vi "rs3 Advanced get color correction3.vi"(8 "error in (no error)":errorcluster, 10 "mode":i32, 11 "device in":u64) -> (0 "error out 2":errorcluster, 1 "error":u64, 2 "STColorCorrection output":T1, 3 "Dev out":u64)   [LabVIEW 2017, in "libRealSense3.lvlib"]
doc: "Opens communication to a specific RealSense Device."
uses:
  libRealSense3.lvlib
  realsense2.dll
panel:
  # "RS3 Adv. Get Color Correct. 2"
  # "(C) 2017 Intel Corp.,  AGJ"
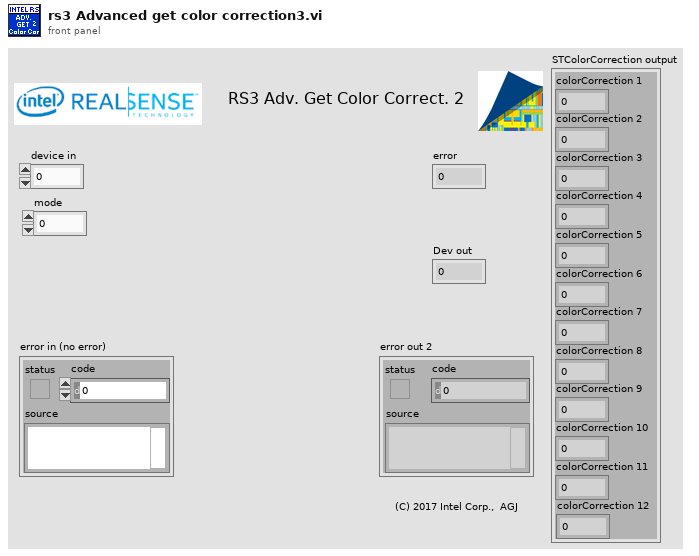
[diagram p1: front panel]
types:
  T1 = cluster{"colorCorrection 1":sgl, "colorCorrection 2":sgl, "colorCorrection 3":sgl, "colorCorrection 4":sgl, "colorCorrection 5":sgl, "colorCorrection 6":sgl, "colorCorrection 7":sgl, "colorCorrection 8":sgl, "colorCorrection 9":sgl, "colorCorrection 10":sgl, "colorCorrection 11":sgl, "colorCorrection 12":sgl}
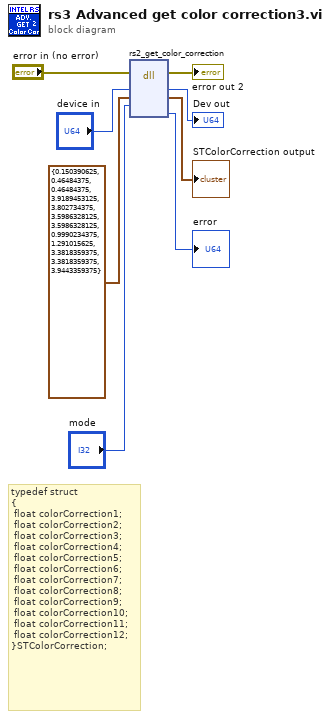
[diagram p0: block diagram]
diagram:
  # "typedef struct\n{\n\tfloat colorCorrection1;\n\tfloat colorCorrection2;\n\tfloat colorCorrection3;\n\tfloat colorCorrection4;\n\tfloat colorCorrection5;\n\tfloat colorCorrection6;\n\tfloat colorCorrection7;\n\tfloat colorCorrection8;\n\tfloat colorCorrection9;\n\tfloat colorCorrection10;\n\tfloat colorCorrection11;\n\tfloat colorCorrection12;\n}STColorCorrection;"
  n1 = dll-call lib="C:/Users/agrunnet/Documents/libRealSense6/realsense2.dll" fn="rs2_get_color_correction"(error in="error in (no error)", "device"="device in", "Color correction"=T1 {"colorCorrection 1"=0.15039062, "colorCorrection 2"=0.46484375, "colorCorrection 3"=0.46484375, "colorCorrection 4"=3.9189453, "colorCorrection 5"=3.8027344, "colorCorrection 6"=3.5986328, "colorCorrection 7"=3.5986328, "colorCorrection 8"=0.99902344, "colorCorrection 9"=1.2910156, "colorCorrection 10"=3.381836, "colorCorrection 11"=3.381836, "colorCorrection 12"=3.944336} ("STColorCorrection input"), "mode"="mode") -> (error out=→"error out 2":errorcluster, "device"=→"Dev out":u64, "Color correction"=→"STColorCorrection output":T1, "error"=→"error":u64)  [unwired: 5 in, 1 out]
